vi "Is Query.vi"(11 "Command in":T1) -> (2 "query?":bool, 3 "Command out":T1)   [LabVIEW 2018, in "Kronos.lvlib" / "Kronos.lvclass"]
uses:
  Kronos.lvclass
  PPLs/Laser/Parent/Laser.lvlibp/Custom Controls/Command List.ctl
  PPLs/Laser/Parent/Laser.lvlibp/Laser.lvclass
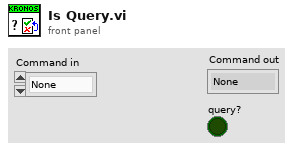
[diagram p1: front panel]
types:
  T1 = typedef "Laser.lvlibp/Laser.lvclass/Command List.ctl" = enum16{"None", "Config?", "Volt?", "ThCase?", "STS?", "Mon?", "Help?", "HB", "Verbose", "Spnt", "Ext", "PRF", "Start", "Stop", "PRF?", "State?", "Status?", "Stat?", "Read HB", "Logon", "Poutmax", "saveconfig", "Reset", "Poutmax?", "PoutCommandMax", "PoutCommandMax?", "FreqMin", "FreqMin?"}
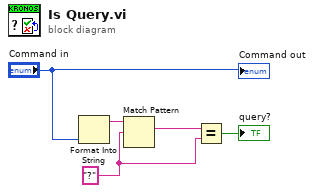
[diagram p0: block diagram]
diagram:
  w3 = "?" ("regular expression")
  n1 = Format Into String("Command in") -> (resulting string=w1:string)  [unwired: 3 in, 1 out]
  n2 = Match Pattern(string=w1, regular expression=w3) -> (match substring=w4:string)  [unwired: 1 in, 3 out]
  n3 = Equal?(x=w4, y=w3) -> (x = y?=→"query?":bool)
  "Command out" <- "Command in"
